vi "Initilize Globals.vi"() -> ()   [LabVIEW 2014]
uses:
  ctt's/Image to Display event.ctt
  <vilib>/vision/Image Controls.llb/IMAQ Image.ctl
  <vilib>/Utility/miscctls.llb/LVRectTypeDef.ctl
panel:
  in  "High Capacity?":bool
  in  "Additional error information":string
  out "Image controller display info":T2(array[cluster])
  out "Display controller Window Bounds":T3={"Left"=0, "Top"=0, "Right"=100, "Bottom"=100}
  in  "Keep mage display controller in corner?":bool=TRUE
  in  "Current window Black/White Levels":cluster{ext, ext}(slide)={1.0, 65535.0} scale=0.0..255.0
  in  "Serial Number for Image Buffers":i32
  in  "Display controller Presets":T4(array[cluster])=[{"Mem"=FALSE, "Black"=-32500.0, "White"=-25000.0, "Recall"=FALSE}]
  in  "Display image event":refnum<user-event>
  in  "Shutter":i32(ring) items=["Auto", "Stay Open", "Always Closed"]
  in  "Number of acquisition blocks":i8(slide)=10 scale=0.0..20.0
  in  "Pixels":cluster{"H Pixels":u32, "V Pixels":u32}
  out "Camera Acquiring":bool
  in  "Image Size":T5={"H Bin"=1024.0, "V Bin"=1024.0, "Left"=1.0, "Right"=1024.0, "Top"=1.0, "Bottom"=1024.0} {"V Bin" min=0.0; "H Bin" min=0.0 step=1.0}
  out "Pixel Size":dbl
  in  "Acquisition Parameters":T6={"Readout Mode"=enum."Image", "Set Acquisition Mode"=enum."Single Scan", "Trigger Mode"=enum."Internal", "Exposure Time (s)"=1.0, "Accumulation Cycle (s)"=0.0, "Kinetic Cycle Time (s)"=1.0, "Number of Kinetics"=1, "Number of Accumulations"=1, "Set VS Speed"=1, "Pixel Rate"=enum."Standard CCD 3 Mhz 14 bits", "V Shift Amplitude"=enum."+1", "Preamp Gain"=enum."1.0"}
  out "Output Amplification":i32
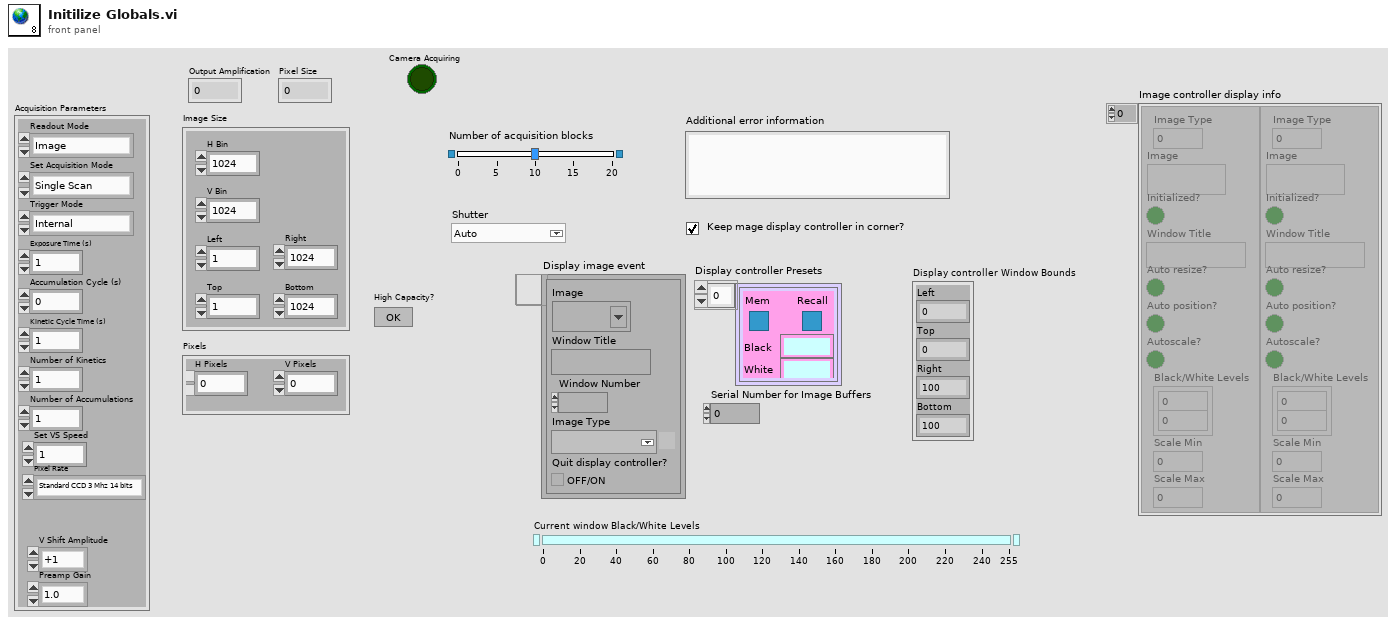
[diagram p1: front panel]
types:
  T1 = typedef "IMAQ Image.ctl" = refnum<image>
  T2 = cluster{"Image Type":u32, "Image":T1, "Initialized?":bool, "Window Title":string, "Auto resize?":bool, "Auto position?":bool, "Autoscale?":bool, "Black/White Levels":cluster{ext, ext}, "Scale Min":ext, "Scale Max":ext}[]
  T3 = typedef "LVRectTypeDef.ctl" = cluster{"Left":i16, "Top":i16, "Right":i16, "Bottom":i16}
  T4 = cluster{"Mem":bool, "Black":ext, "White":ext, "Recall":bool}[]
  T5 = cluster{"H Bin":dbl, "V Bin":dbl, "Left":dbl, "Right":dbl, "Top":dbl, "Bottom":dbl}
  T6 = cluster{"Readout Mode":enum16{"Full Vertical Binning", "Multi-Track", "Random-Track", "Single-Track", "Image"}, "Set Acquisition Mode":enum16{"(do nothing)", "Single Scan", "Accumulate", "Kinetics", "Fast Kinetics", "Run till abort"}, "Trigger Mode":enum16{"Internal", "External"}, "Exposure Time (s)":dbl, "Accumulation Cycle (s)":dbl, "Kinetic Cycle Time (s)":dbl, "Number of Kinetics":i32, "Number of Accumulations":i32, "Set VS Speed":i32, "Pixel Rate":enum16{"EM CCD 10 Mhz 14 bits", "EM CCD 5 Mhz 14 bits", "EM CCD 3 Mhz 14 bits", "EM CCD 1 Mhz 16 bits", "Standard CCD 3 Mhz 14 bits", "Standard CCD 1 Mhz 16 bits"}, "V Shift Amplitude":enum16{"normal", "+1", "+2", "+3", "+4"}, "Preamp Gain":enum16{"1.0", "2.4", "5.0"}}
diagram:
